vi "CC Parse Declination.vi"(8 "error in (no error)":errorcluster, 11 "Declination string":string) -> (0 "error out":errorcluster, 2 "Angle":dbl, 3 "Declination":T1)   [LabVIEW 2024]
uses:
  Telescope/Telescope cluster Declination.ctl
  <vilib>/regexp/Match Regular Expression.xnode
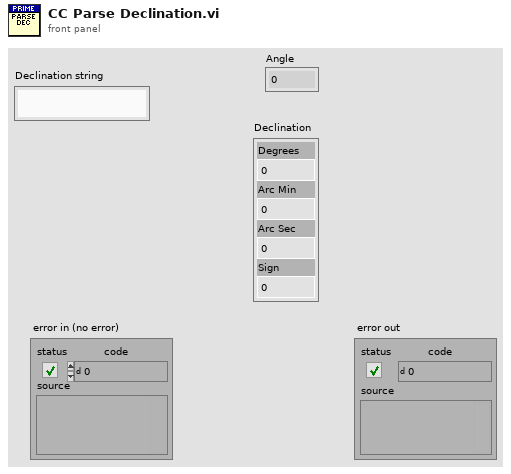
[diagram p1: front panel]
types:
  T1 = typedef "Telescope cluster Declination.ctl" = cluster{"Degrees":dbl, "Arc Min":dbl, "Arc Sec":dbl, "Sign":dbl}
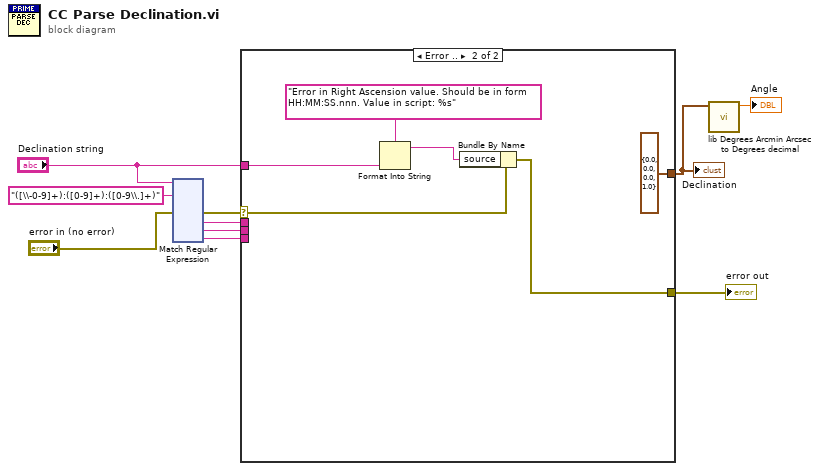
[diagram p0: block diagram]
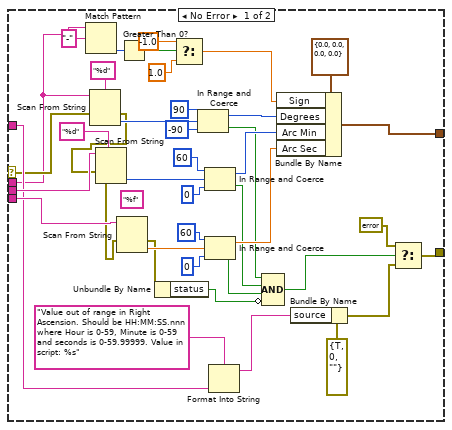
[diagram p2: hidden frame]
diagram:
  n1 = xnode "Match Regular Expression"("input string"="Declination string", "regular expression"="([\\-0-9]+):([0-9]+):([0-9\\.]+)", "error in"="error in (no error)") -> ("error out"=w5:errorcluster, "submatch 1"=w9:string, "submatch 2"=w8:string, "submatch 3"=w7:string)  [unwired: 3 in, 4 out]
  n2 = case shown="Error .." w5 {
    selector: w5 -> [w23 w55]
    tunnel: w9 -> [w17 _]
    tunnel: w8 -> [w49 _]
    tunnel: w7 -> [w48 _]
    tunnel: [w35 T1 {"Degrees"=0.0, "Arc Min"=0.0, "Arc Sec"=0.0, "Sign"=1.0} ("Declination")] -> w2
    tunnel: "Declination string" -> [w26 w56]
    tunnel: [w24 w53] -> w3
    frame No Error {
      (unwired) "%f" ("format string")
      n3 = Match Pattern(string=w17, regular expression="-") -> (offset past match=w16:i32)  [unwired: 1 in, 3 out]
      n4 = Scan From String(format string="%d", input string=w17, error in=w23) -> (error out=w22:errorcluster, output 1=w47:i32)  [unwired: 2 in, 2 out]
      n5 = Scan From String(format string="%d", input string=w49, error in=w22) -> (error out=w21:errorcluster, output 1=w44:i32)  [unwired: 2 in, 2 out]
      n6 = Scan From String(input string=w48, error in=w21) -> (error out=w20:errorcluster, output 1=w39:dbl)  [unwired: 3 in, 2 out]
      n7 = Greater Than 0?(x=w16) -> (x > 0?=w15:bool)
      n8 = Unbundle By Name(w20) -> ("status"=w19:bool)
      n9 = Select(t=-1.0, s=w15, f=1.0 ("t")) -> (s? t:f=w12:dbl)
      n10 = In Range and Coerce(upper limit=90, x=w47, lower limit=-90) -> (coerced(x)=w38:i32, In Range?=w34:bool)
      n11 = In Range and Coerce(upper limit=60, x=w44, lower limit=0) -> (coerced(x)=w37:i32, In Range?=w33:bool)
      n12 = In Range and Coerce(upper limit=60, x=w39, lower limit=0) -> (coerced(x)=w36:dbl, In Range?=w32:bool)
      n13 = Format Into String(format string="Value out of range in Right Ascension. Should be HH:MM:SS.nnn where Hour is 0-59, Minute is 0-59 and seconds is 0-59.99999. Value in script: %s", w26) -> (resulting string=w25:string)  [unwired: 2 in, 1 out]
      n14 = Compound Arithmetic op=AND(w34, w33, w32, invert w19) -> (w31:bool)
      n15 = Bundle By Name(cluster=T1 {"Degrees"=0.0, "Arc Min"=0.0, "Arc Sec"=0.0, "Sign"=0.0} ("Declination"), "Sign"=w12, "Degrees"=w38, "Arc Min"=w37, "Arc Sec"=w36) -> (w35:T1)
      n16 = Bundle By Name(cluster=errorcluster {"status"=TRUE, "code"=0, "source"=""} ("error out"), "source"=w25) -> (w29:errorcluster)
      n17 = Select(t=errorcluster {"status"=FALSE, "code"=0, "source"=""}, s=w31, f=w29) -> (s? t:f=w24:errorcluster)
    }
    frame Error {
      n18 = Format Into String(format string="Error in Right Ascension value. Should be in form HH:MM:SS.nnn. Value in script: %s", w56) -> (resulting string=w54:string)  [unwired: 2 in, 1 out]
      n19 = Bundle By Name(cluster=w55, "source"=w54) -> (w53:errorcluster)
    }
  }
  "error out" <- w3
  "Declination" <- w2
  n20 = call "lib Degrees Arcmin Arcsec to Degrees decimal.vi"("Declination"=w2) -> ("Angle"=→"Angle":dbl)  [unwired: 9 in, 1 out]
